vi "FindChessboardCornersSectorBasedARGB.vi"(5 "Flags (Default - None)":T2[](array[typedef]), 7 "Chessboard Corners Info":T4, 8 "error in (no error)":errorcluster, 11 "ARGB Image in":T5) -> (0 "error out":errorcluster, 1 "Meta Data":T1[][](array[typedef]), 2 "Points":T3[](array[typedef]), 3 "ARGB Image":T5)   [LabVIEW 2020, in "feature_detection.lvlib"]
doc: "Detect the Chessboard in the Image and return the <b>Internal</b> Corner Points."
uses:
  feature_detection.lvlib
  image/ARGB Image.ctl
  Chessboard Corner Info.ctl
  common/Image Point (Float).ctl
  Find Chessboard Corners Sector Based Flags.ctl
  Find Chessboard Corners Sector Based Meta.ctl
  6a9761e7-0504-45a6-89a0-1e961674e9fc.vi
  <vilib>/Utility/error.llb/Error Cluster From Error Code.vi
  common/common.lvlib
  image/image.lvlib
panel:
  # "Note: See this issue on the behaviour of this function\n\nhttps://github.com/opencv/opencv/issues/22083"
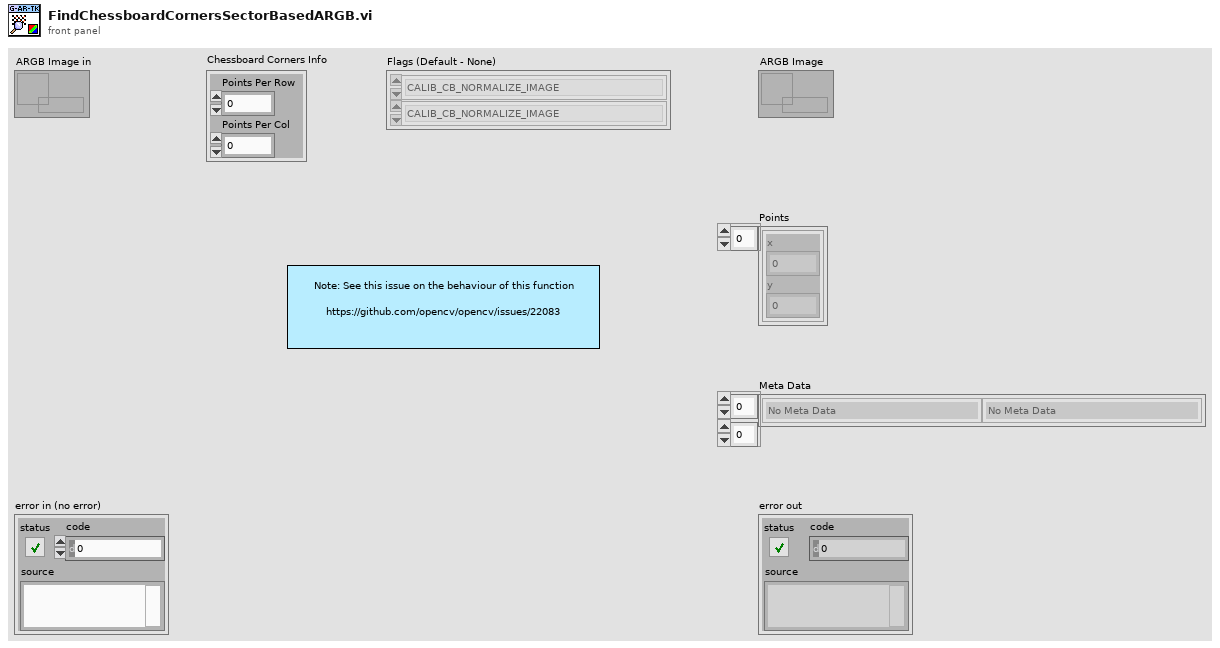
[diagram p1: front panel]
types:
  T1 = typedef "feature_detection.lvlib/Find Chessboard Corners Sector Based Meta.ctl" = enum16{"No Meta Data", "Left-Top Corner Black Cell", "Left-Top Corner White Cell", "Left-Top Corner Black Cell with Marker", "Left-Top Corner White Cell with Marker"}
  T2 = typedef "feature_detection.lvlib/Find Chessboard Corners Sector Based Flags.ctl" = enum16{"CALIB_CB_NORMALIZE_IMAGE", "CALIB_CB_EXHAUSTIVE", "CALIB_CB_ACCURACY", "CALIB_CB_LARGER", "CALIB_CB_MARKER"}
  T3 = typedef "common.lvlib/Image Point (Float).ctl" = cluster{"x":dbl, "y":dbl}
  T4 = typedef "feature_detection.lvlib/Chessboard Corner Info.ctl" = cluster{"Points Per Row":u8, "Points Per Col":u8}
  T5 = typedef "image.lvlib/ARGB Image.ctl" = refnum<data-value>
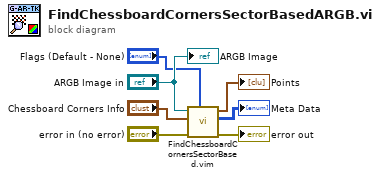
[diagram p0: block diagram]
diagram:
  n1 = call "FindChessboardCornersSectorBased.vim"("Flags (Default - None)"="Flags (Default - None)", "error in (no error)"="error in (no error)", "Chessboard Corners Info"="Chessboard Corners Info", "Src"="ARGB Image in") -> ("error out"=→"error out":errorcluster, "Meta Data"=→"Meta Data":T1[][], "Points"=→"Points":T3[])  [unwired: 5 in]
  "ARGB Image" <- "ARGB Image in"
